vi "prePurge2.vi"(8 "error in":errorcluster, 9 "Boiler Simulation Controls":refnum<vi>, 10 "Boiler Controls":refnum<vi>, 11 "Boiler Status Indicators":refnum<vi>) -> (0 "error out":errorcluster, 3 "elapsedTime":dbl)   [LabVIEW 2024]
uses:
  Controls/Boiler Simulation Controls.ctl
  Controls/Boiler Status Indicators.ctl
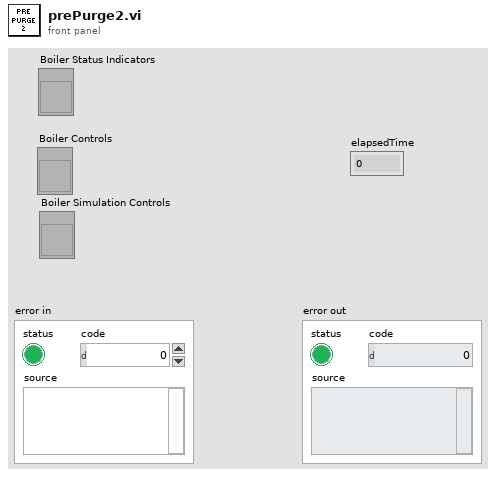
[diagram p1: front panel]
types:
  T1 = typedef "Boiler Status Indicators.ctl" = cluster{"Status":string, "Primary Fan":bool, "Natural Gas Valve":bool, "Pilot":bool, "Fuel Valve":bool, "Forced Draft Fan":bool, "Time Count":dbl}
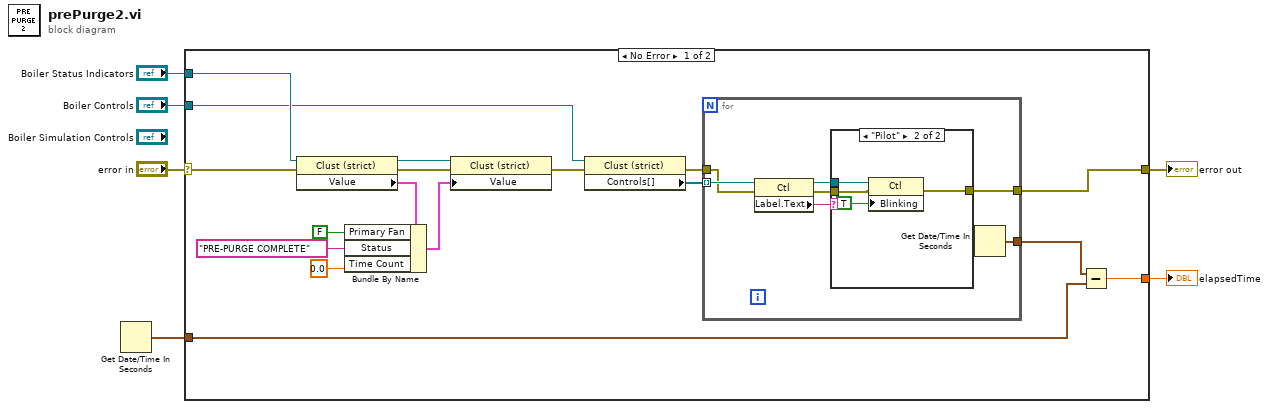
[diagram p0: block diagram]
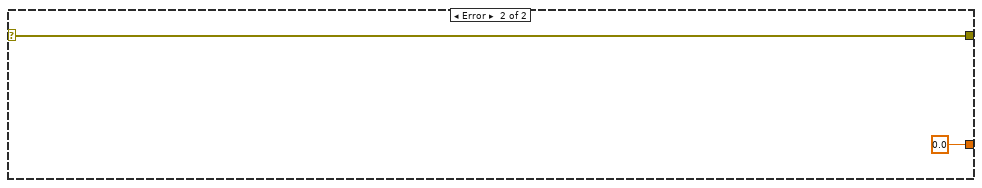
[diagram p3: hidden frame]
diagram:
  n1 = Get Date/Time In Seconds() -> (seconds since 1Jan1904=w3:timestamp)
  n2 = case shown="No Error" "error in" {
    selector: "error in" -> [w23 w37]
    tunnel: [w11 w37] -> w5
    tunnel: "Boiler Status Indicators" -> [w22 _]
    tunnel: w3 -> [w10 _]
    tunnel: [w9 0.0] -> w2
    tunnel: "Boiler Controls" -> [w7 _]
    frame No Error {
      n3 = property class="Clust (strict)"(reference=w22, error in=w23) -> (reference out=w21:refnum<vi>, error out=w20:errorcluster, "Value"=w19:T1)
      n4 = Bundle By Name(cluster=w19, "Primary Fan"=FALSE, "Status"="PRE-PURGE COMPLETE", "Time Count"=0.0) -> (w18:T1)
      n5 = property class="Clust (strict)"(reference=w21, error in=w20, "Value"=w18) -> (error out=w14:errorcluster)  [unwired: 1 out]
      n6 = property class="Clust (strict)"(reference=w7, error in=w14) -> (error out=w12:errorcluster, "Controls[]"=w13:refnum<vi>[])  [unwired: 1 out]
      n7 = for {
        tunnel: w13 -> [w30] mode=indexing
        tunnel: w12 -> [w28]
        tunnel: [w25] -> w11
        tunnel: [w24] -> w8
        n8 = property class="Ctl"(reference=w30, error in=w28) -> (reference out=w27:refnum<vi>, error out=w26:errorcluster, "Label.Text"=w29:string)
        n9 = case shown="\"Pilot\"" w29 {
          tunnel: w27 -> [_ w35]
          tunnel: w26 -> [w31 w34]
          tunnel: [w31 w32] -> w25
          frame "False", Default {
          }
          frame "Pilot" {
            n10 = property class="Ctl"(reference=w35, error in=w34, "Blinking"=TRUE) -> (error out=w32:errorcluster)  [unwired: 1 out]
          }
        }
        n11 = Get Date/Time In Seconds() -> (seconds since 1Jan1904=w24:timestamp)
      }
      n12 = Subtract(x=w8, y=w10) -> (x-y=w9:dbl)
    }
    frame Error {
    }
  }
  "error out" <- w5
  "elapsedTime" <- w2
